vi "errorToXmlString.vi"(8 "error in (no error)":errorcluster) -> (0 "error out":errorcluster, 2 "xmlString":string, 3 "XmlParser out":refnum<class "XmlParser.lvclass">)   [LabVIEW 2011, in "Tools.lvlib" / "xml.lvlib" / "XmlParser.lvclass"]
uses:
  XmlParser.lvclass
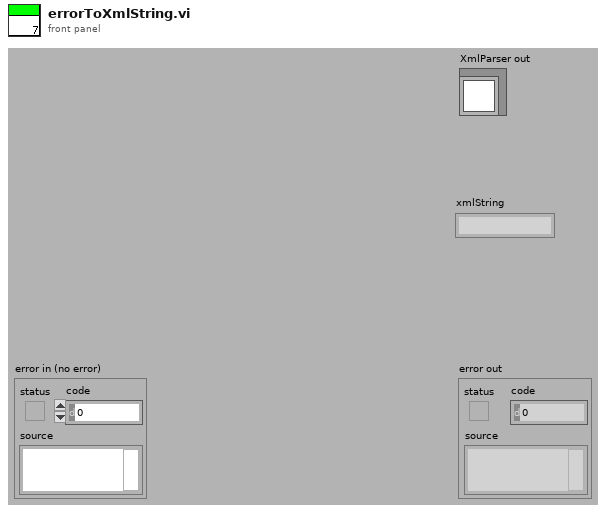
[diagram p1: front panel]
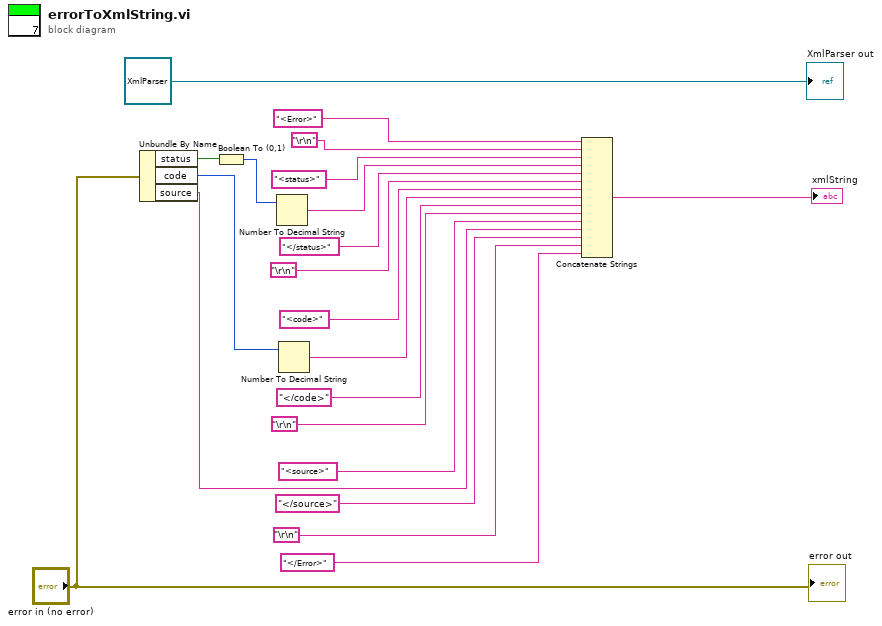
[diagram p0: block diagram]
diagram:
  n1 = Unbundle By Name("error in (no error)") -> ("status"=w16:bool, "code"=w9:i32, "source"=w5:string)
  n2 = Boolean To (0,1)(Boolean=w16) -> (0, 1=w15:i16)
  n3 = Number To Decimal String(number=w15) -> (decimal integer string=w14:string)  [unwired: 1 in]
  n4 = Number To Decimal String(number=w9) -> (decimal integer string=w10:string)  [unwired: 1 in]
  n5 = Concatenate Strings("<Error>", "\r\n", "<status>", w14, "</status>", "\r\n", "<code>", w10, "</code>", "\r\n", "<source>", w5, "</source>", "\r\n", "</Error>") -> (→"xmlString":string)
  "error out" <- "error in (no error)"
  "XmlParser out" <- refnum<class "XmlParser.lvclass"> refnum ("XmlParser in")
